vi "Get OS Architecture.vi"(8 "error in (no error)":errorcluster) -> (0 "error out":errorcluster, 2 "found?":bool, 3 "OS architecture":enum16{"32-bit", "64-bit"}(ring))   [LabVIEW 2013]
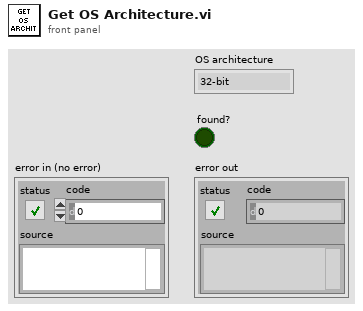
[diagram p1: front panel]
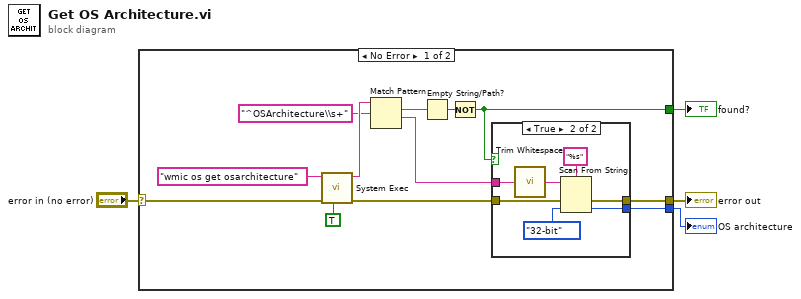
[diagram p0: block diagram]
diagram:
  n1 = case shown="No Error" "error in (no error)" {
    selector: "error in (no error)" -> [w8 w25]
    tunnel: [w5 _] -> w4
    tunnel: [w7 w25] -> w3
    tunnel: [w6 _] -> w1
    frame No Error {
      n2 = call <vilib>:"System Exec.vi"("run minimized? (F)"=TRUE, "error in (no error)"=w8, "command line"="wmic os get osarchitecture") -> ("error out"=w9:errorcluster, "standard output"=w14:string)  [unwired: 5 in, 2 out]
      n3 = Match Pattern(string=w14, regular expression="^OSArchitecture\\s+") -> (match substring=w11:string, after substring=w12:string)  [unwired: 1 in, 2 out]
      n4 = Empty String/Path?(string/path=w11) -> (empty?=w10:bool)
      n5 = Not(x=w10) -> (.not. x?=w5:bool)
      n6 = case shown="True" w5 {
        tunnel: w12 -> [_ w24]
        tunnel: w9 -> [w17 w23]
        tunnel: [w17 w22] -> w7
        tunnel: [_ w18] -> w6
        frame False {
        }
        frame True {
          n7 = call <vilib>:"Trim Whitespace.vi"("string"=w24) -> ("trimmed string"=w21:string)  [unwired: 1 in]
          n8 = Scan From String(format string="%s", input string=w21, error in=w23, default 1=enum16{"32-bit", "64-bit"}."32-bit") -> (error out=w22:errorcluster, output 1=w18:enum16{"32-bit", "64-bit"})  [unwired: 1 in, 2 out]
        }
      }
    }
    frame Error {
    }
  }
  "found?" <- w4
  "error out" <- w3
  "OS architecture" <- w1
